vi "GetChannelMeas.vi"(0 "VISA IN":refnum<visa-resource-name>="GPIB1::16::INSTR", 5 "error in":errorcluster) -> (14 "VISA Out":refnum<visa-resource-name>="GPIB1::16::INSTR", 19 "error out":errorcluster={"status"=TRUE, "code"=-1074001424, "source"="BlkXfer.vi -> Instrument Error: 106: +106,\"Requested measurement not found\""})   [LabVIEW 2018, in "PNA-X.lvlib"]
uses:
  PNA-X.lvlib
panel:
  out "chndata":dbl[][](graph)
  out "ChnData":dbl[][](array[numeric])
  out "Msemnts":string[](array[string])
  out "FileNames":string[](array[string])
  in  "Channel":i32=1
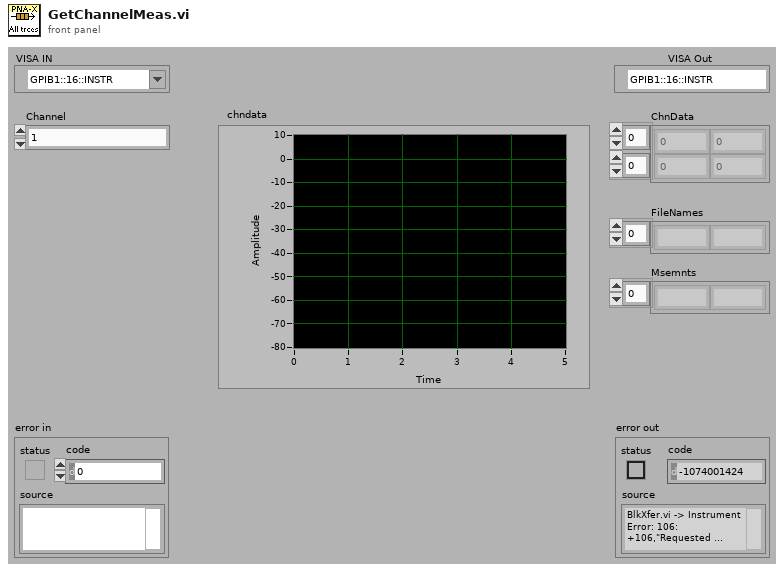
[diagram p1: front panel]
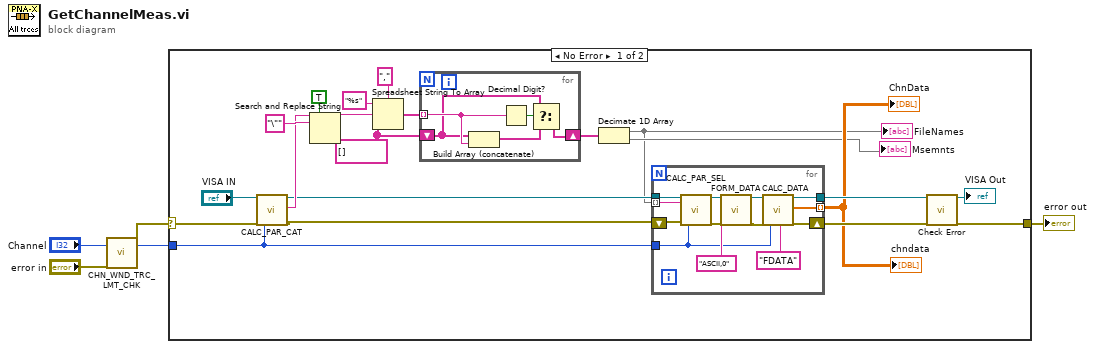
[diagram p0: block diagram]
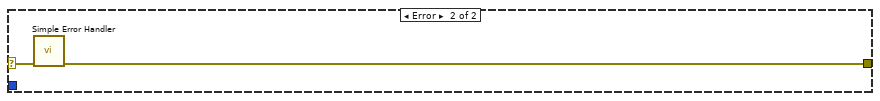
[diagram p2: hidden frame]
diagram:
  n1 = call "CHN_WND_TRC_LMT_CHK.vi"("Channel"="Channel", "error in"="error in") -> ("error out"=w3:errorcluster, "Channel"=w2:i32)  [unwired: 13 in, 3 out]
  n2 = case shown="No Error" w3 {
    selector: w3 -> [w23 w46]
    tunnel: [w26 w45] -> w4
    tunnel: w2 -> [w16 _]
    frame No Error {
      w9 = string[] []
      n3 = call "CALC_PAR_CAT.vi"("VISA IN"="VISA IN", "error in"=w23, "Channel"=w16) -> ("VISA Out"=w14:refnum<visa-resource-name>, "Data"=w20:string, "error out"=w15:errorcluster)  [unwired: 12 in, 2 out]
      n4 = Search and Replace String(replace all?=TRUE ("replace all? (F)"), input string=w20, search string="\"") -> (result string=w19:string)  [unwired: 5 in, 3 out]
      n5 = Spreadsheet String To Array(delimiter (Tab)="," ("regular expression"), format string="%s", spreadsheet string=w19, array type (2D Dbl)=w9) -> (array=w10:string[])
      n6 = for {
        tunnel: w10 -> [w30] mode=indexing
        shift-right: [w27] -> w8
        shift-left: w9 -> [w28]
        n7 = Build Array (concatenate)(w28, w30) -> (w29:string[])
        n8 = Decimal Digit?(1:w30) -> (0:w31:bool)
        n9 = Select(t=w28, s=w31, f=w29) -> (s? t:f=w27:string[])
      }
      n10 = Decimate 1D Array(w8) -> (w6:string[], →"Msemnts":string[])
      "FileNames" <- w6
      n11 = for {
        tunnel: w16 -> [w38]
        tunnel: w14 -> [w36]
        shift-right: [w35] -> w12
        shift-left: w15 -> [w37]
        tunnel: [w34] -> w11 mode=indexing
        tunnel: [w33] -> w13
        tunnel: w6 -> [w32] mode=indexing
        n12 = call "CALC_PAR_SEL.vi"("VISA IN"=w36, "Measurement"=w32, "error in"=w37, "Channel"=w38) -> ("VISA Out"=w44:refnum<visa-resource-name>, "error out"=w43:errorcluster)  [unwired: 14 in]
        n13 = call "FORM_DATA.vi"("VISA IN"=w44, "error in"=w43, "DataType"="ASCII,0") -> ("VISA Out"=w40:refnum<visa-resource-name>, "error out"=w41:errorcluster)  [unwired: 15 in]
        n14 = call "CALC_DATA.vi"("VISA IN"=w40, "error in"=w41, "Channel"=w38, "DataType"="FDATA") -> ("VISA Out"=w33:refnum<visa-resource-name>, "array"=w34:dbl[], "error out"=w35:errorcluster)  [unwired: 13 in]
      }
      "ChnData" <- w11
      "chndata" <- w11
      n15 = call "Check Error.vi"("VISA Resource Name"=w13, "error in (no error)"=w12) -> ("dup VISA session"=→"VISA Out":refnum<visa-resource-name>, "error out"=w26:errorcluster)  [unwired: 16 in]
    }
    frame Error {
      n16 = call <vilib>:"Simple Error Handler.vi"("error in (no error)"=w46) -> ("error out"=w45:errorcluster)  [unwired: 4 in, 4 out]
    }
  }
  "error out" <- w4
